vi "band_filter.vi"(2 "hi_freq":dbl format="%.2f", 3 "low_Freq":dbl format="%.2f", 4 "df":dbl format="%.2f", 5 "In":dbl[](array[numeric]) format="%.2f") -> (0 "PWR_BAND":dbl format="%.2f", 1 "Out":dbl[](array[numeric]) format="%.2f")   [LabVIEW 2013]
panel:
  out "XY Graph":cluster{dbl[], dbl[]}(graph)
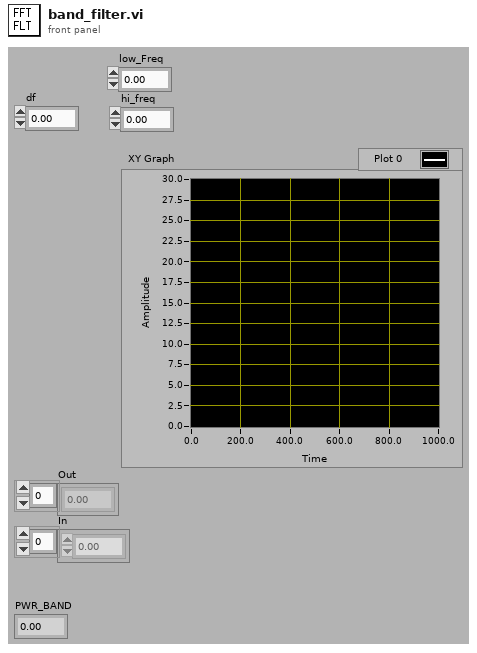
[diagram p1: front panel]
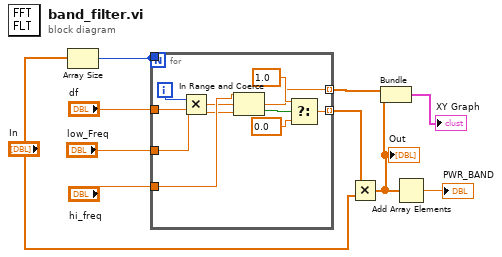
[diagram p0: block diagram]
diagram:
  n1 = Array Size(array="In") -> (size(s)=w2:i32)
  n2 = for {
    N: w2 -> [_]
    tunnel: "df" -> [w14]
    tunnel: w2 -> [_]
    tunnel: [w16] -> w5 mode=indexing
    tunnel: "hi_freq" -> [w13]
    tunnel: "low_Freq" -> [w12]
    tunnel: [w11] -> w6 mode=indexing
    i -> [w15]
    n3 = Multiply(x=w15, y=w14) -> (x*y=w11:dbl)
    n4 = In Range and Coerce(upper limit=w13, x=w11, lower limit=w12) -> (In Range?=w19:bool)  [unwired: 1 out]
    n5 = Select(t=1.0, s=w19, f=0.0) -> (s? t:f=w16:dbl)
  }
  n6 = Multiply(x=w5, y="In") -> (x*y=w3:dbl[])
  "Out" <- w3
  n7 = Bundle(w6, w3) -> (→"XY Graph":cluster{dbl[], dbl[]})  [unwired: 1 in]
  n8 = Add Array Elements(numeric array=w3) -> (sum=→"PWR_BAND":dbl)
